vi "Week1_Exercise1.vi"() -> ()   [LabVIEW 2015]
panel:
  in  "stop":bool
  out "Boolean":bool
  out "Thermometer":dbl(slide) scale=0.0..100.0
  out "Gauge":dbl(knob) scale=0.0..10.0
  out "Meter":dbl(knob) scale=0.0..10.0
  out "Numeric 2":dbl
  in  "Knob":dbl(knob) scale=0.0..10.0
  in  "Slide 2":dbl(slide) scale=0.0..10.0
  in  "Slide":dbl(slide) scale=0.0..10.0
  in  "Numeric":dbl
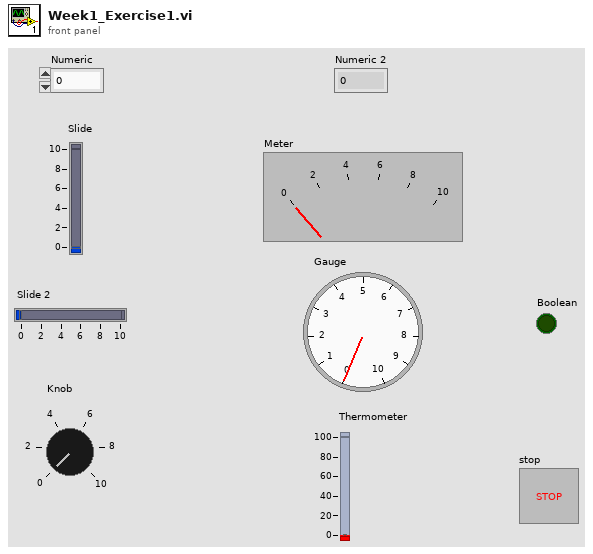
[diagram p1: front panel]
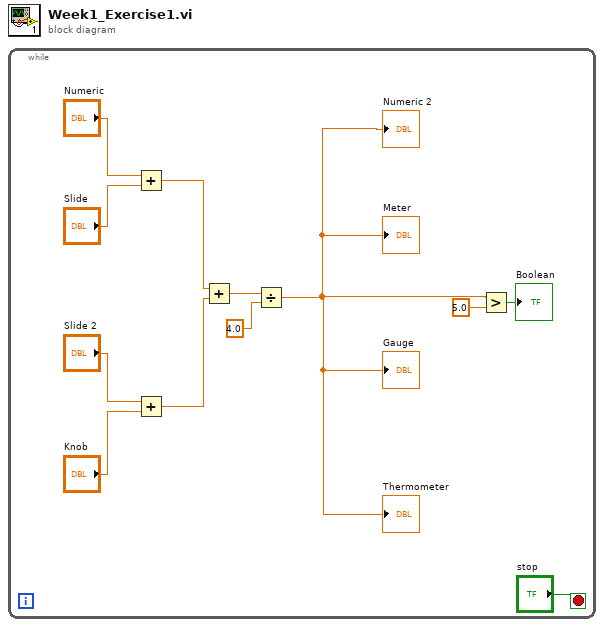
[diagram p0: block diagram]
diagram:
  n1 = while {
    stop <- "stop" stop-if-true
    n2 = Add(x="Numeric", y="Slide") -> (x+y=w8:dbl)
    n3 = Add(x="Slide 2", y="Knob") -> (x+y=w7:dbl)
    n4 = Add(x=w8, y=w7) -> (x+y=w3:dbl)
    n5 = Divide(x=w3, y=4.0) -> (x/y=w1:dbl)
    "Numeric 2" <- w1
    "Meter" <- w1
    "Gauge" <- w1
    "Thermometer" <- w1
    n6 = Greater?(x=w1, y=5.0) -> (0:→"Boolean":bool)
  }
